vi "Create Sysdef Tree from DB Channel Clusters_BC_Create Description.vi"(6 "Word Index":i32, 7 "Type":enum16{"DW", "STC", "SPC", "SW", "TI", "AC"}(ring), 8 "error in (no error)":errorcluster, 9 "Message Name":string, 10 "CWD1":T1, 11 "messageType":T2) -> (0 "error out":errorcluster, 3 "Description (Out)":string)   [LabVIEW 2020, in "Ballard 1553 System Explorer.lvlib"]
uses:
  Ballard 1553 System Explorer.lvlib
  Parse XML Ballard/Ballard_messageType.ctl
  Parse XML Ballard/Ballard_CWD1.ctl
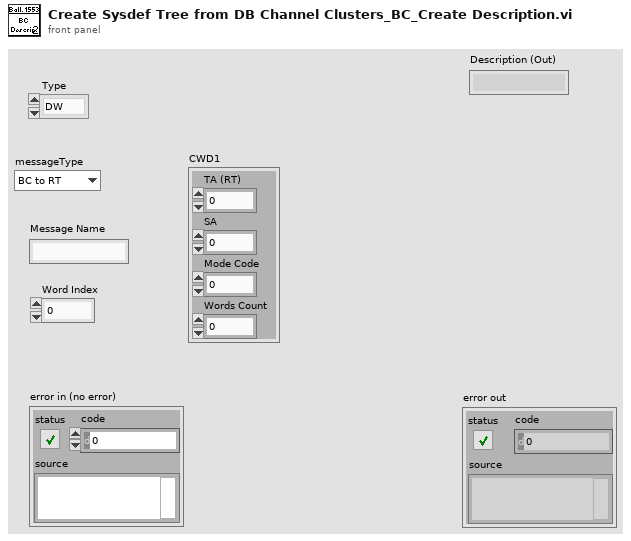
[diagram p1: front panel]
types:
  T1 = typedef "Ballard 1553 System Explorer.lvlib/Ballard_CWD1.ctl" = cluster{"TA (RT)":i8, "SA":i8, "Mode Code":i8, "Words Count":i8}
  T2 = typedef "Ballard 1553 System Explorer.lvlib/Ballard_messageType.ctl" = enum16{"BC to RT", "RT to BC", "RT to RT", "MC (Rx)", "MC (Tx)"}
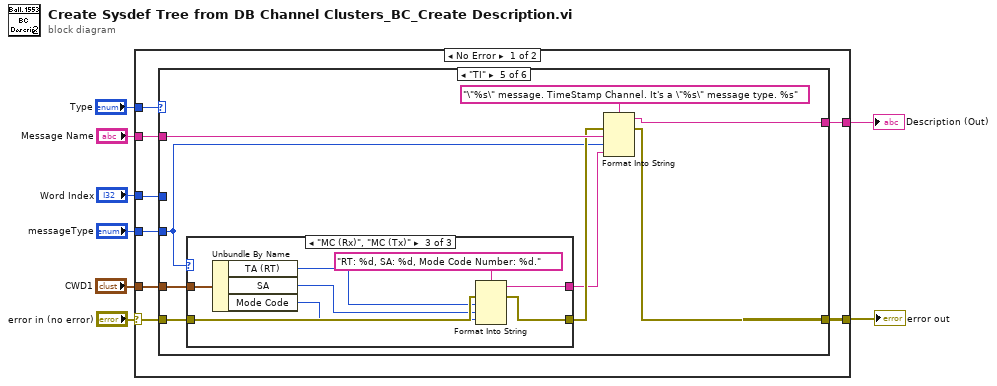
[diagram p0: block diagram]
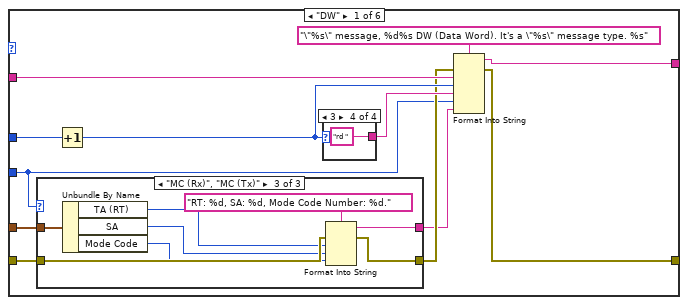
[diagram p2: hidden frame]
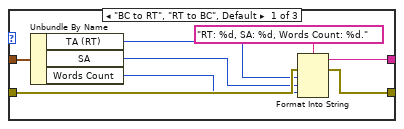
[diagram p3: hidden frame]
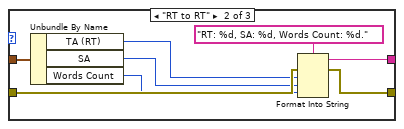
[diagram p4: hidden frame]
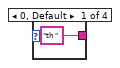
[diagram p5: hidden frame]
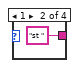
[diagram p6: hidden frame]
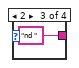
[diagram p7: hidden frame]
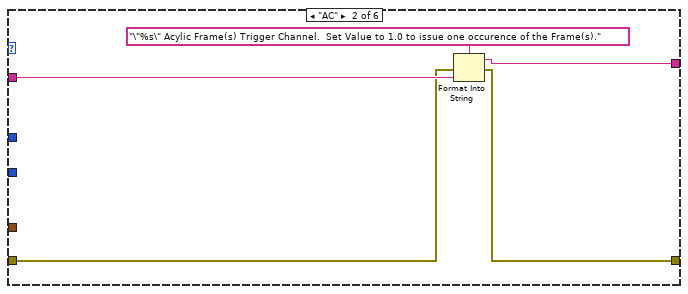
[diagram p8: hidden frame]
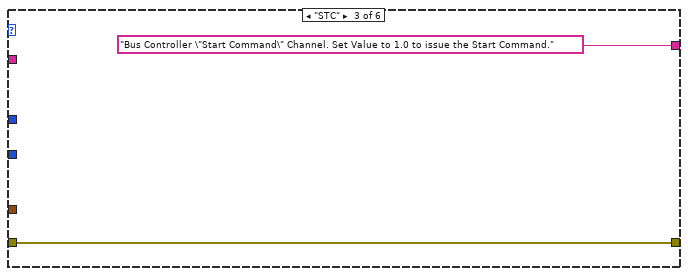
[diagram p9: hidden frame]
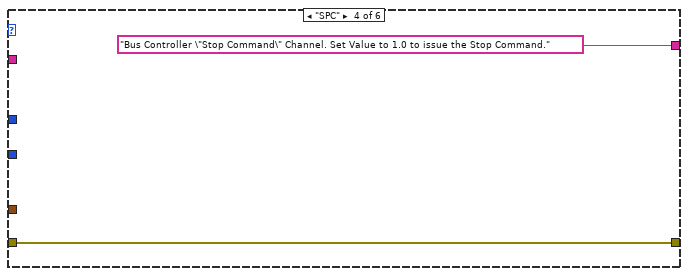
[diagram p10: hidden frame]
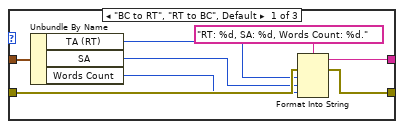
[diagram p11: hidden frame]
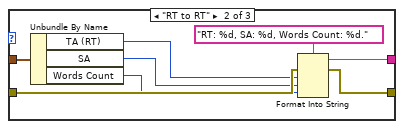
[diagram p12: hidden frame]
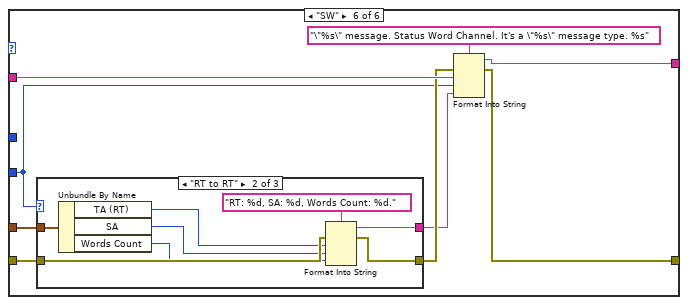
[diagram p13: hidden frame]
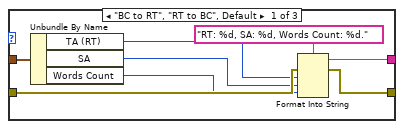
[diagram p14: hidden frame]
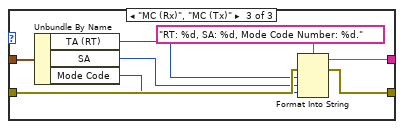
[diagram p15: hidden frame]
diagram:
  n1 = case shown="No Error" "error in (no error)" {
    selector: "error in (no error)" -> [w11 w132]
    tunnel: [w16 w132] -> w7
    tunnel: "Message Name" -> [w15 _]
    tunnel: "messageType" -> [w13 _]
    tunnel: "Word Index" -> [w14 _]
    tunnel: "CWD1" -> [w12 _]
    tunnel: [w10 _] -> w2
    tunnel: "Type" -> [w9 _]
    frame No Error {
      n2 = case shown="\"TI\"" w9 {
        tunnel: [w28 w61 w63 w65 w74 w107] -> w16
        tunnel: w15 -> [w27 w60 _ _ w73 w106]
        tunnel: w14 -> [w25 _ _ _ _ _]
        tunnel: w13 -> [w17 _ _ _ w67 w100]
        tunnel: w12 -> [w22 _ _ _ w71 w104]
        tunnel: w11 -> [w21 w57 w63 w65 w70 w103]
        tunnel: [w18 w58 "Bus Controller \"Start Command\" Channel. Set Value to 1.0 to issue the Start Command." "Bus Controller \"Stop Command\" Channel. Set Value to 1.0 to issue the Stop Command." w68 w101] -> w10
        frame "DW" {
          n3 = case shown="\"MC (Rx)\", \"MC (Tx)\"" w17 {
            tunnel: w22 -> [w34 w42 w50]
            tunnel: w21 -> [w36 w44 w52]
            tunnel: [w35 w43 w51] -> w20
            tunnel: [w29 w37 w45] -> w19
            frame "BC to RT", "RT to BC", Default {
              n4 = Unbundle By Name(w34) -> ("TA (RT)"=w33:i8, "SA"=w32:i8, "Words Count"=w31:i8)
              n5 = Format Into String(format string="RT: %d, SA: %d, Words Count: %d.", error in=w36, w33, w32, w31) -> (resulting string=w29:string, error out=w35:errorcluster)  [unwired: 1 in]
            }
            frame "RT to RT" {
              n6 = Unbundle By Name(w42) -> ("TA (RT)"=w41:i8, "SA"=w40:i8, "Words Count"=w39:i8)
              n7 = Format Into String(format string="RT: %d, SA: %d, Words Count: %d.", error in=w44, w41, w40, w39) -> (resulting string=w37:string, error out=w43:errorcluster)  [unwired: 1 in]
            }
            frame "MC (Rx)", "MC (Tx)" {
              n8 = Unbundle By Name(w50) -> ("TA (RT)"=w49:i8, "SA"=w48:i8, "Mode Code"=w47:i8)
              n9 = Format Into String(format string="RT: %d, SA: %d, Mode Code Number: %d.", error in=w52, w49, w48, w47) -> (resulting string=w45:string, error out=w51:errorcluster)  [unwired: 1 in]
            }
          }
          n10 = Increment(x=w25) -> (x+1=w24:i32)
          n11 = case shown="3" w24 {
            tunnel: ["th " "st " "nd " "rd "] -> w23
            frame 0, Default {
            }
            frame 1 {
            }
            frame 2 {
            }
            frame 3 {
            }
          }
          n12 = Format Into String(format string="\"%s\" message, %d%s DW (Data Word). It's a \"%s\" message type. %s", error in=w20, w27, w24, w23, w17, w19) -> (resulting string=w18:string, error out=w28:errorcluster)  [unwired: 1 in]
        }
        frame "AC" {
          n13 = Format Into String(format string="\"%s\" Acylic Frame(s) Trigger Channel.  Set Value to 1.0 to issue one occurence of the Frame(s).", error in=w57, w60) -> (resulting string=w58:string, error out=w61:errorcluster)  [unwired: 1 in]
        }
        frame "STC" {
        }
        frame "SPC" {
        }
        frame "TI" {
          n14 = case shown="\"MC (Rx)\", \"MC (Tx)\"" w67 {
            tunnel: w71 -> [w80 w88 w96]
            tunnel: w70 -> [w82 w90 w98]
            tunnel: [w81 w89 w97] -> w69
            tunnel: [w75 w83 w91] -> w66
            frame "BC to RT", "RT to BC", Default {
              n15 = Unbundle By Name(w80) -> ("TA (RT)"=w79:i8, "SA"=w78:i8, "Words Count"=w77:i8)
              n16 = Format Into String(format string="RT: %d, SA: %d, Words Count: %d.", error in=w82, w79, w78, w77) -> (resulting string=w75:string, error out=w81:errorcluster)  [unwired: 1 in]
            }
            frame "RT to RT" {
              n17 = Unbundle By Name(w88) -> ("TA (RT)"=w87:i8, "SA"=w86:i8, "Words Count"=w85:i8)
              n18 = Format Into String(format string="RT: %d, SA: %d, Words Count: %d.", error in=w90, w87, w86, w85) -> (resulting string=w83:string, error out=w89:errorcluster)  [unwired: 1 in]
            }
            frame "MC (Rx)", "MC (Tx)" {
              n19 = Unbundle By Name(w96) -> ("TA (RT)"=w95:i8, "SA"=w94:i8, "Mode Code"=w93:i8)
              n20 = Format Into String(format string="RT: %d, SA: %d, Mode Code Number: %d.", error in=w98, w95, w94, w93) -> (resulting string=w91:string, error out=w97:errorcluster)  [unwired: 1 in]
            }
          }
          n21 = Format Into String(format string="\"%s\" message. TimeStamp Channel. It's a \"%s\" message type. %s", error in=w69, w73, w67, w66) -> (resulting string=w68:string, error out=w74:errorcluster)  [unwired: 1 in]
        }
        frame "SW" {
          n22 = case shown="\"RT to RT\"" w100 {
            tunnel: w104 -> [w113 w121 w129]
            tunnel: w103 -> [w115 w123 w131]
            tunnel: [w114 w122 w130] -> w102
            tunnel: [w108 w116 w124] -> w99
            frame "BC to RT", "RT to BC", Default {
              n23 = Unbundle By Name(w113) -> ("TA (RT)"=w112:i8, "SA"=w111:i8, "Words Count"=w110:i8)
              n24 = Format Into String(format string="RT: %d, SA: %d, Words Count: %d.", error in=w115, w112, w111, w110) -> (resulting string=w108:string, error out=w114:errorcluster)  [unwired: 1 in]
            }
            frame "RT to RT" {
              n25 = Unbundle By Name(w121) -> ("TA (RT)"=w120:i8, "SA"=w119:i8, "Words Count"=w118:i8)
              n26 = Format Into String(format string="RT: %d, SA: %d, Words Count: %d.", error in=w123, w120, w119, w118) -> (resulting string=w116:string, error out=w122:errorcluster)  [unwired: 1 in]
            }
            frame "MC (Rx)", "MC (Tx)" {
              n27 = Unbundle By Name(w129) -> ("TA (RT)"=w128:i8, "SA"=w127:i8, "Mode Code"=w126:i8)
              n28 = Format Into String(format string="RT: %d, SA: %d, Mode Code Number: %d.", error in=w131, w128, w127, w126) -> (resulting string=w124:string, error out=w130:errorcluster)  [unwired: 1 in]
            }
          }
          n29 = Format Into String(format string="\"%s\" message. Status Word Channel. It's a \"%s\" message type. %s", error in=w102, w106, w100, w99) -> (resulting string=w101:string, error out=w107:errorcluster)  [unwired: 1 in]
        }
      }
    }
    frame Error {
    }
  }
  "error out" <- w7
  "Description (Out)" <- w2
